vi "load cor.vi"(8 "error in (no error)":errorcluster, 11 "filename":string) -> (0 "error out":errorcluster, 3 "function return":i16)   [LabVIEW 2015, in "SCANalone4x64.lvlib"]
doc: "__declspec(dllimport) short __stdcall load_cor(const char* filename);"
uses:
  <userlib>/SCANalone4x64/SCANalone4x64.lvlib
  <userlib>/SCANalone4x64/SCANalone4x64.dll
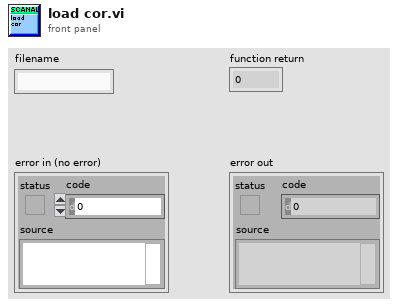
[diagram p1: front panel]
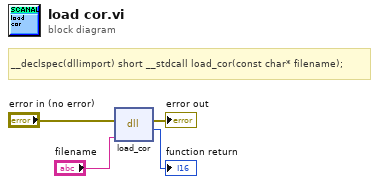
[diagram p0: block diagram]
diagram:
  # "__declspec(dllimport) short __stdcall load_cor(const char* filename);"
  n1 = dll-call lib="C:/Program Files/National Instruments/LabVIEW 2015/user.lib/SCANalone4x64/SCANalone4x64.*" fn="load_cor"(error in="error in (no error)", "filename"="filename") -> (error out=→"error out":errorcluster, →"function return":i16)  [unwired: 3 in, 1 out]
